vi "Pressure-Voltage.vi"() -> ()   [LabVIEW 2015]
uses:
  <vilib>/Utility/error.llb/DialogType.ctl
  <vilib>/DAQmx/read.llb/DAQmx Read (Analog DBL 1Chan 1Samp).vi
  <vilib>/DAQmx/create/channels.llb/DAQmx Create Channel (AI-Voltage-Basic).vi
  <vilib>/DAQmx/miscellaneous.llb/DAQmx Fill In Error Info.vi
panel:
  in  "stop":bool
  out "Slide":dbl(slide)=0.444662221506717 scale=0.0..1.0
  out "output variable":dbl=0.444662221506717
  out "Gauge":dbl(knob)=0.444662221506717 scale=0.0..1.0
  out "Waveform Chart":dbl(graph)=0.444662221506717
  out "Vi 2":dbl=0.7398038924745398 format="%0.2f"
  out "Vi":dbl=0.7398038924745398 format="%0.2f"
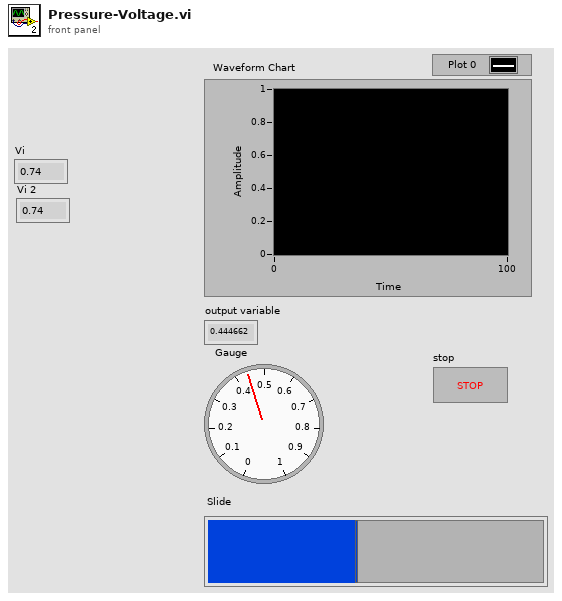
[diagram p1: front panel]
types:
  T1 = typedef "DialogType.ctl" = u16
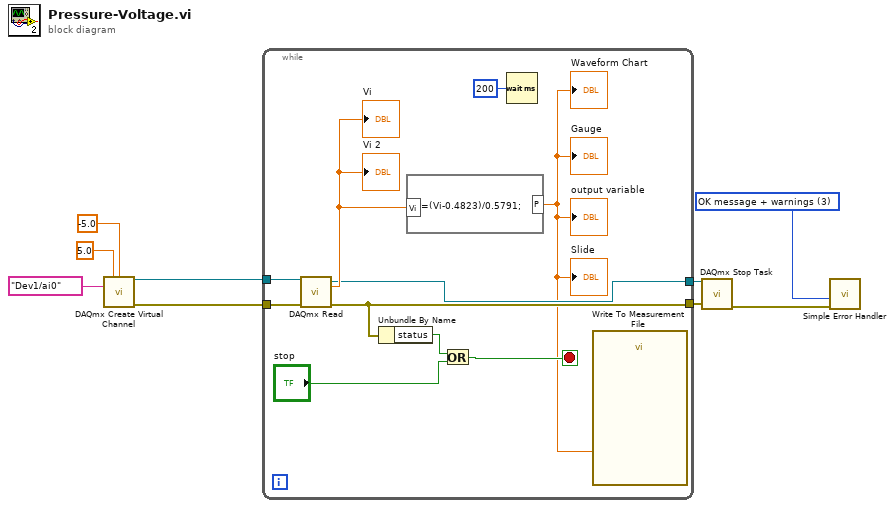
[diagram p0: block diagram]
diagram:
  w1 = T1 3 items=["no dialog", "OK message", "continue or stop message", "OK message + warnings", "continue/stop + warnings"] ("type of dialog (OK msg:1)")
  n1 = call-poly <vilib>:"DAQmx Create Virtual Channel.vi"("maximum value"=5.0, "minimum value"=-5.0, "physical channels"=tag "Dev1/ai0") -> ("task out"=w6:refnum<k21>, "error out"=w5:errorcluster)  [unwired: 11 in]
  n2 = while {
    tunnel: w6 -> [w19]
    tunnel: w5 -> [w18]
    tunnel: [w16] -> w4
    tunnel: [w12] -> w3
    stop <- w13 stop-if-true
    n3 = call-poly <vilib>:"DAQmx Read.vi"("task/channels in"=w19, "error in"=w18) -> ("task out"=w12:refnum<k21>, "data"=w17:dbl, "error out"=w16:errorcluster)  [unwired: 11 in]
    "Vi" <- w17
    "Vi 2" <- w17
    n4 = Unbundle By Name(w16) -> ("status"=w15:bool)
    n5 = formula code="P=(Vi-0.4823)/0.5791;"("Vi"=w17) -> ("P"=w10:dbl)
    "Waveform Chart" <- w10
    "Gauge" <- w10
    "output variable" <- w10
    "Slide" <- w10
    n6 = Or(x=w15, y="stop") -> (x .or. y?=w13:bool)
    n7 = Wait (ms)(milliseconds to wait=u32 200) -> ()  [unwired: 1 out]
    n8 = call "Write To Measurement File"("Signals"=w10) -> ()  [unwired: 16 in, 3 out]
  }
  n9 = call <vilib>:"DAQmx Stop Task.vi"("task/channels in"=w3, "error in"=w4) -> ("error out"=w2:errorcluster)  [unwired: 12 in, 1 out]
  n10 = call <vilib>:"Simple Error Handler.vi"("type of dialog (OK msg:1)"=w1, "error in (no error)"=w2) -> ()  [unwired: 3 in, 5 out]
